vi "Example Kafka Write Events Data.vi"() -> ()   [LabVIEW 2019]
doc: "This example demonstrates how to write measured data along with text and timestamp values to a .tdms file using the TDMS API. TDMS files written by this example can be read by the example TDMS Read Events Data.vi."
panel:
  in  "Stop":bool
  out "Measured Data":waveform(dbl)[](graph)
  # "Overview: Demonstrates the use of the TDMS Write function to write measured data along with text and timestamp values to a .tdms file.\nInstructions:\n1. Run the VI.\n2. Click Stop to stop the VI.\n3. Open the TDMS Read Events Data.vi example to view the data generated by this VI."
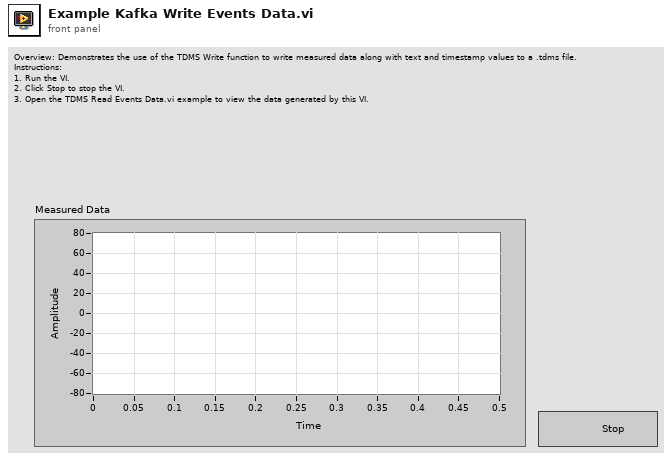
[diagram p1: front panel]
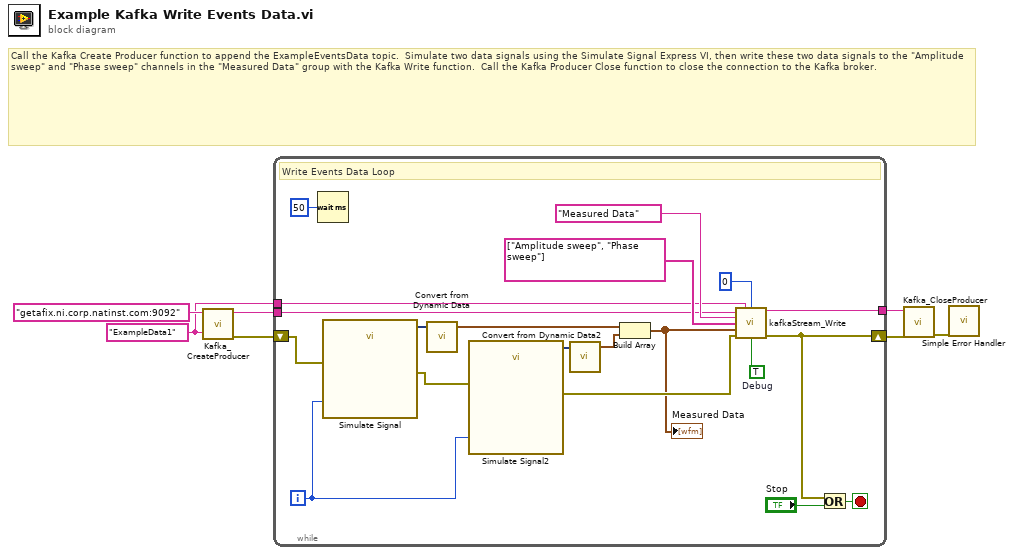
[diagram p0: block diagram]
diagram:
  w2 = "ExampleData1" ("Topic")
  # "Call the Kafka Create Producer function to append the ExampleEventsData topic.  Simulate two data signals using the Simulate Signal Express VI, then write these two data signals to the \"Amplitude sweep\" and \"Phase sweep\" channels in the \"Measured Data\" group with the Kafka Write function.  Call the Kafka Producer Close function to close the connection to the Kafka broker."
  n1 = call "Kafka_CreateProducer.vi"("Topic"=w2, "Kafka Broker"="getafix.ni.corp.natinst.com:9092") -> ("error out"=w5:errorcluster, "Producer Handle"=w6:string)  [unwired: 8 in]
  n2 = while {
    shift-right: [w9] -> w4
    shift-left: w5 -> [w24]
    tunnel: w6 -> [w13]
    tunnel: [w12] -> w3
    tunnel: w2 -> [w11]
    i -> [w21]
    stop <- w25 stop-if-true
    w8 = TRUE  # Debug
    # "Write Events Data Loop"
    n3 = Wait (ms)(milliseconds to wait=u32 50) -> ()  [unwired: 1 out]
    n4 = call "Simulate Signal"("Amplitude"=w21, "error in (no error)"=w24) -> ("Sine"=w23:dynamicdata, "error out"=w22:errorcluster)  [unwired: 12 in]
    n5 = call "Convert from Dynamic Data"("Dynamic Data Type"=w23) -> ("Waveform"=w18:waveform(dbl))  [unwired: 3 in]
    n6 = call "Simulate Signal2"("Phase"=w21, "error in (no error)"=w22) -> ("Sine"=w20:dynamicdata, "error out"=w17:errorcluster)  [unwired: 12 in]
    n7 = call "Convert from Dynamic Data2"("Dynamic Data Type"=w20) -> ("Waveform"=w19:waveform(dbl))  [unwired: 3 in]
    n8 = Build Array(w18, w19) -> (w16:waveform(dbl)[])
    "Measured Data" <- w16
    n9 = call "kafkaStream_Write.vi"("Kafka Producer Handle"=w13, "File Name"=w11, "Kafka Partition"=u32 0, "Group Name"="Measured Data" ("group name"), "Channel Names"=string[] ["Amplitude sweep", "Phase sweep"] ("channel names"), "Waveforms"=w16, "error in (no error)"=w17, "Debug"=w8) -> ("Kafka Producer Handle Out"=w12:string, "error out"=w9:errorcluster)  [unwired: 3 in, 3 out]
    n10 = Or(x=w9, y="Stop") -> (x .or. y?=w25:bool)
  }
  n11 = call "Kafka_CloseProducer.vi"("error in (no error)"=w4, "Producer Handle"=w3) -> ("error out"=w1:errorcluster)  [unwired: 8 in, 1 out]
  n12 = call <vilib>:"Simple Error Handler.vi"("error in (no error)"=w1) -> ()  [unwired: 2 in, 7 out]
